vi "interpolation of X-tether by Volt-tether and stuckbead scan.vi"(2 "stuckbead-QPD (V)":dbl[](array[numeric]), 4 "stuckbead-stage position (um)":dbl[](array[numeric]), 5 "tether-QPD (V)":dbl[](array[numeric])) -> (1 "Xt-interpolated (um)":dbl[](array[numeric]))   [LabVIEW 2014]
panel:
  out "Vt":dbl
  out "Vs2":dbl
  out "Vs1":dbl
  out "Xs2":dbl
  out "Xs1":dbl
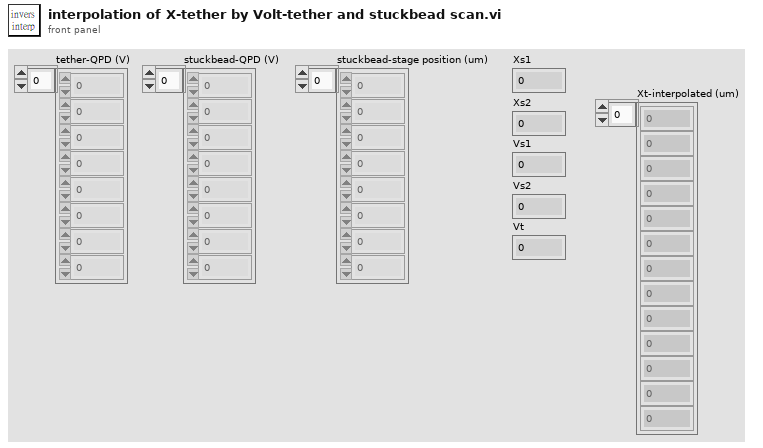
[diagram p1: front panel]
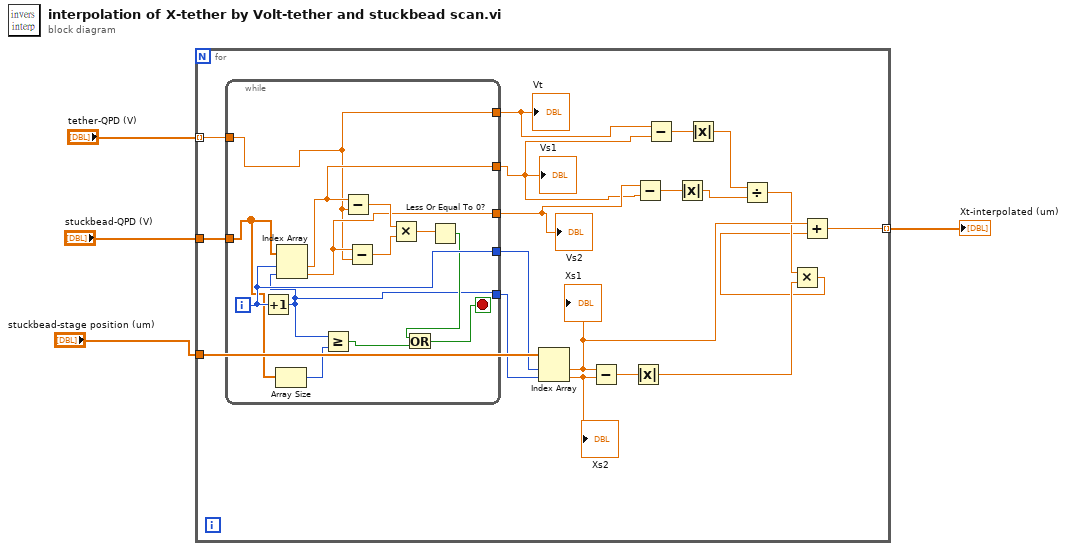
[diagram p0: block diagram]
diagram:
  n1 = for {
    tunnel: "stuckbead-QPD (V)" -> [w23]
    tunnel: "tether-QPD (V)" -> [w22] mode=indexing
    tunnel: "stuckbead-stage position (um)" -> [w21]
    tunnel: [w5] -> w1 mode=indexing
    n2 = while {
      tunnel: w23 -> [w27]
      tunnel: [w33] -> w19
      tunnel: [w28] -> w18
      tunnel: w22 -> [w30]
      tunnel: [w32] -> w11
      tunnel: [w31] -> w12
      tunnel: [w30] -> w13
      i -> [w33]
      stop <- w24 stop-if-true
      n3 = Increment(x=w33) -> (x+1=w28:i32)
      n4 = Array Size(array=w27) -> (size(s)=w26:i32)
      n5 = Index Array(array=w27, index #1=w33, index #2=w28) -> (element #1=w32:dbl, element #2=w31:dbl)
      n6 = Greater Or Equal?(x=w28, y=w26) -> (x >= y?=w25:bool)
      n7 = Subtract(x=w32, y=w30) -> (x-y=w36:dbl)
      n8 = Subtract(x=w31, y=w30) -> (x-y=w35:dbl)
      n9 = Multiply(x=w36, y=w35) -> (x*y=w34:dbl)
      n10 = Less Or Equal To 0?(x=w34) -> (x <= 0?=w29:bool)
      n11 = Or(x=w29, y=w25) -> (x .or. y?=w24:bool)
    }
    "Vs1" <- w11
    "Vs2" <- w12
    "Vt" <- w13
    n12 = Index Array(array=w21, index #1=w19, index #2=w18) -> (element #1=w16:dbl, element #2=w17:dbl)
    "Xs1" <- w16
    "Xs2" <- w17
    n13 = Subtract(x=w16, y=w17) -> (x-y=w20:dbl)
    n14 = Absolute Value(x=w20) -> (abs(x)=w8:dbl)
    n15 = Subtract(x=w12, y=w11) -> (x-y=w15:dbl)
    n16 = Subtract(x=w13, y=w11) -> (x-y=w14:dbl)
    n17 = Absolute Value(x=w15) -> (abs(x)=w9:dbl)
    n18 = Absolute Value(x=w14) -> (abs(x)=w10:dbl)
    n19 = Divide(x=w10, y=w9) -> (x/y=w7:dbl)
    n20 = Multiply(x=w7, y=w8) -> (x*y=w6:dbl)
    n21 = Add(x=w16, y=w6) -> (x+y=w5:dbl)
  }
  "Xt-interpolated (um)" <- w1
